vi "Config Layer Count.vi"(5 "Trigger Count (1)":u32=1, 7 "Arm Count (1)":u32=1, 8 "error in":errorcluster, 9 "Channel (Channel A)":T1, 10 "Node In":string, 11 "VISA resource name":refnum<visa-resource-name>) -> (0 "error out":errorcluster, 2 "Node Out":string, 3 "VISA resource name out":refnum<visa-resource-name>, 4 "Command String":string)   [LabVIEW 2013, in "Keithley 2600 Series.lvlib"]
doc: "This VI sets the number of times the SMU should iterate through the arm and trigger layers during a sweep.\n\n<b>Functions and Attributes Used</b>\nsmuX.trigger.arm.count\nsmuX.trigger.count"
uses:
  Keithley 2600 Series.lvlib
  Private/GlobalVariables.vi
  Channel.ctl
panel:
  # "(c) 2008 Keithley Instruments, Inc.  ALL RIGHTS RESERVED."
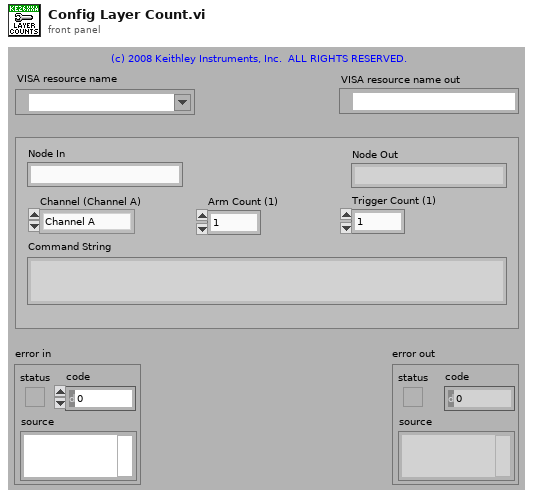
[diagram p1: front panel]
types:
  T1 = typedef "Keithley 2600 Series.lvlib/Channel.ctl" = enum32{"Channel A", "Channel B"}
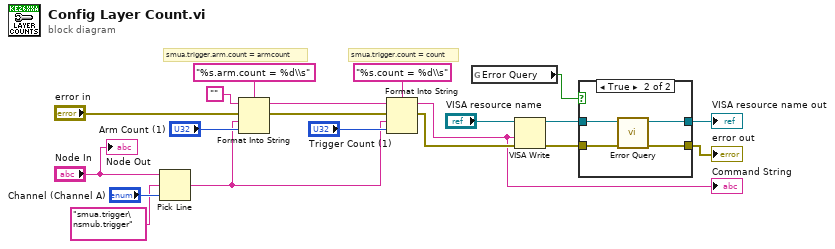
[diagram p0: block diagram]
diagram:
  # "smua.trigger.count = count"
  # "smua.trigger.arm.count = armcount"
  n1 = Pick Line(string ("")="Node In", multi-line string="smua.trigger\nsmub.trigger", line index="Channel (Channel A)") -> (output string=w11:string)
  n2 = Format Into String(format string="%s.arm.count = %d\\s", initial string="", error in="error in", w11, "Arm Count (1)") -> (resulting string=w9:string, error out=w14:errorcluster)
  n3 = Format Into String(format string="%s.count = %d\\s", initial string=w9, error in=w14, w11, "Trigger Count (1)") -> (resulting string=w1:string, error out=w8:errorcluster)
  "Command String" <- w1
  n4 = global read "GlobalVariables.vi" "Error Query"() -> (w6:bool)
  n5 = VISA Write(VISA resource name="VISA resource name", write buffer=w1, error in (no error)=w8) -> (VISA resource name out=w5:refnum<visa-resource-name>, error out=w4:errorcluster)  [unwired: 1 out]
  n6 = case shown="True" w6 {
    tunnel: w5 -> [w22 w26]
    tunnel: w4 -> [w21 w25]
    tunnel: [w22 w24] -> w3
    tunnel: [w21 w23] -> w2
    frame False {
    }
    frame True {
      n7 = call "Error Query.vi"("error in (no error)"=w25, "VISA resource name"=w26) -> ("error out"=w23:errorcluster, "VISA resource name out"=w24:refnum<visa-resource-name>)  [unwired: 8 out]
    }
  }
  "VISA resource name out" <- w3
  "error out" <- w2
  "Node Out" <- "Node In"
